vi "Set Rate (RPM).vi"(8 "error in (no error)":errorcluster, 10 "Rate (RPM)":dbl, 11 "Dev Motors with Brake in":refnum<class "Dev Motors with Brake.lvclass">) -> (0 "error out":errorcluster, 3 "Dev Motors with Brake out":refnum<class "Dev Motors with Brake.lvclass">)   [LabVIEW 2014, in "Dev Motors with Brake.lvlib" / "Dev Motors with Brake.lvclass"]
uses:
  Dev Motors with Brake.lvclass
  Comp Robot/Comp Motors with Encoders/Comp Motors with Encoders Class/Comp Motors with Encoders.lvclass
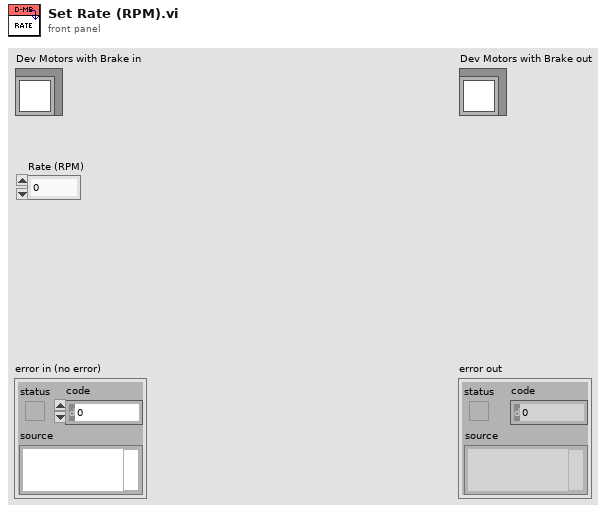
[diagram p1: front panel]
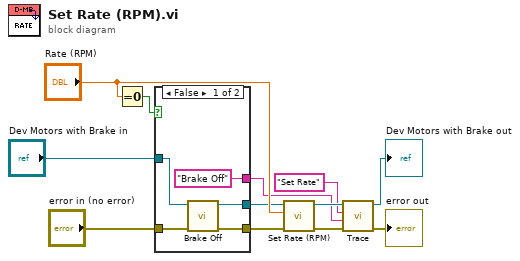
[diagram p0: block diagram]
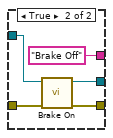
[diagram p2: hidden frame]
diagram:
  n1 = Equal To 0?(x="Rate (RPM)") -> (x = 0?=w1:bool)
  n2 = case shown="False" w1 {
    tunnel: "Dev Motors with Brake in" -> [w17 w22]
    tunnel: [w16 w21] -> w10
    tunnel: "error in (no error)" -> [w15 w19]
    tunnel: [w14 w18] -> w8
    tunnel: ["Brake Off" "Brake Off"] -> w2
    frame False {
      n3 = call-dynamic "Brake Off.vi"("error in (no error)"=w15, "Dev Motors with Brake in"=w17) -> ("error out"=w14:errorcluster, "Dev Motors with Brake out"=w16:refnum<class "Dev Motors with Brake.lvclass">)  [unwired: 8 in]
    }
    frame True {
      n4 = call-dynamic "Brake On.vi"("error in (no error)"=w19, "Dev Motors with Brake in"=w22) -> ("error out"=w18:errorcluster, "Dev Motors with Brake out"=w21:refnum<class "Dev Motors with Brake.lvclass">)  [unwired: 8 in]
    }
  }
  n5 = call-parent "Set Rate (RPM).vi"("error in (no error)"=w8, "Rate (RPM)"="Rate (RPM)", "Comp Motors with Encoders in"=w10) -> ("error out"=w7:errorcluster, "Comp Motors with Encoders out"=w5:refnum<class "Dev Motors with Brake.lvclass">)  [unwired: 7 in]
  n6 = call-dynamic "Trace.vi"("error in (no error)"=w7, "System Message"=w2, "System Action"="Set Rate", "System Actor in"=w5) -> ("error out"=→"error out":errorcluster, "System Actor out"=→"Dev Motors with Brake out":refnum<class "Dev Motors with Brake.lvclass">)  [unwired: 6 in]
